vi "Lvi Subsystem Set Ctr One Shot Repeat Mode.vi"(7 "Polarity":u32, 8 "error in (no error)":errorcluster, 9 "GateEdge":u32, 10 "Millisecs":dbl, 11 "TaskRef":i32) -> (0 "error out":errorcluster, 1 "function return":u32(ring), 2 "ActualMillisecs":dbl, 3 "TaskRef out":i32)   [LabVIEW 2022 SP3, in "DtLvLink.lvlib"]
doc: "Calls directly into the entry points of the DLL of the Data Acq SDK to create one or more virtual channels, add them to a task, and configure the task with the specified settings to output a single pulse for a specified duration (in milliseconds) each time that the device detects a trigger (determined by the counter/timer's gate input signal). This VI is used by the higher-level VI, DtOLCreateTask."
uses:
  DtLvLink.lvlib
  <userlib>/LV-Link3/DtLvLink_64.dll
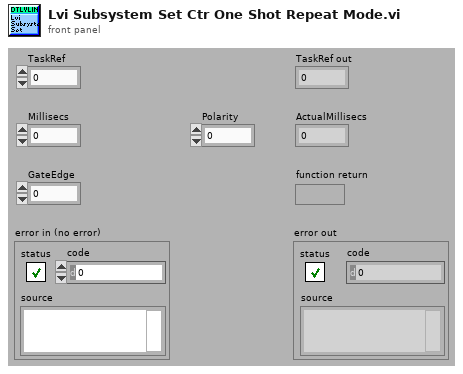
[diagram p1: front panel]
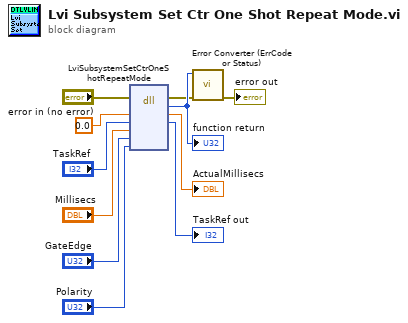
[diagram p0: block diagram]
diagram:
  n1 = dll-call lib="C:/Program Files/National Instruments/LabVIEW 2022/user.lib/LV-Link3/DtLvLink_64.*" fn="LviSubsystemSetCtrOneShotRepeatMode"(error in="error in (no error)", "ActualMillisecs"=0.0, "TaskRef"="TaskRef", "Millisecs"="Millisecs", "GateEdge"="GateEdge", "Polarity"="Polarity") -> (error out=w2:errorcluster, w11:u32, "ActualMillisecs"=→"ActualMillisecs":dbl, "TaskRef"=→"TaskRef out":i32)  [unwired: 5 in, 1 out]
  "function return" <- w11
  n2 = call "Error Converter (ErrCode or Status).vi"("error in (no error)"=w2, "error code"=w11) -> ("error out"=→"error out":errorcluster)  [unwired: 9 in]
